vi "chaos crest close.vi"(11 "connectionHandle":u32) -> (2 "nok":i32, 3 "connectionHandle out":u32)   [LabVIEW 2014, in "libcommon-crest.lvlib"]
doc: "int chaos_crest_close(chaos_crest_handle_t h);"
uses:
  libcommon-crest.lvlib
  chaos-i686-dynamic-release/lib/libcommon-crest.so
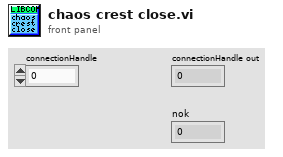
[diagram p1: front panel]
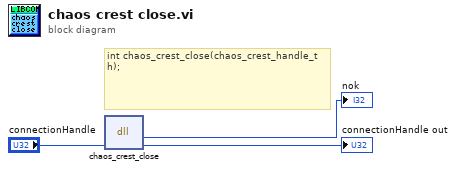
[diagram p0: block diagram]
diagram:
  # "int chaos_crest_close(chaos_crest_handle_t h);"
  n1 = dll-call lib="home/chaos/chaos_bundle/chaos-i686-dynamic-release/lib/libcommon-crest.*" fn="chaos_crest_close"("connectionHandle"="connectionHandle") -> (→"nok":i32, "connectionHandle"=→"connectionHandle out":u32)  [unwired: 3 in, 2 out]
